vi "getValue.vi"(8 "error in (no error)":errorcluster, 11 "type.ImageData in":refnum<class "type.ImageData.lvclass">) -> (0 "error out":errorcluster, 2 "value":variant, 3 "type.ImageData out":refnum<class "type.ImageData.lvclass">)   [LabVIEW 2015, in "type.ImageData.lvclass"]
uses:
  type.ImageData.lvclass
  type.ImageData.lvclass/type.ImageData.ctl
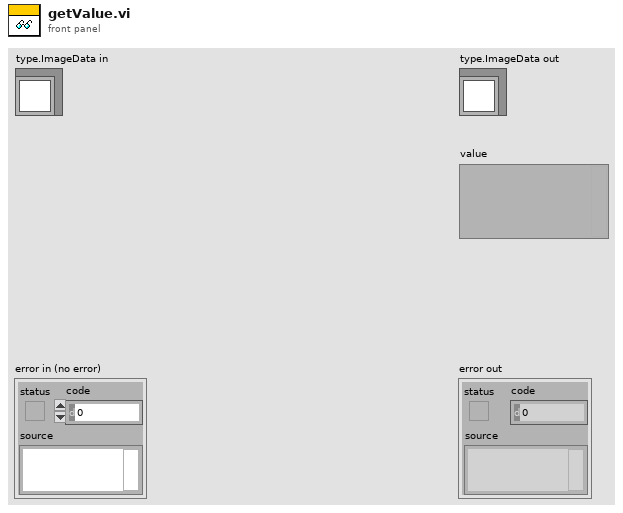
[diagram p1: front panel]
types:
  T1 = typedef "imagedata.ctl" = cluster{"image type":i32, "image depth":i32, "image":u8[], "mask":u8[], "colors":u32[], "Rectangle":cluster{"left":i16, "top":i16, "right":i16, "bottom":i16}}
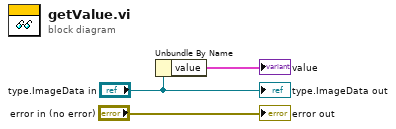
[diagram p0: block diagram]
diagram:
  n1 = Unbundle By Name("type.ImageData in") -> ("value"=→"value":T1)
  "error out" <- "error in (no error)"
  "type.ImageData out" <- "type.ImageData in"
